vi "Connection.vi"(6 "Parameters":variant, 7 "Timeout":i32=5000, 8 "error in (no error)":errorcluster, 9 "Port":u16=102, 10 "IP Address":string, 11 "Simulated_PLC in":refnum<class "Simulated_PLC.lvclass">) -> (0 "error out":errorcluster, 3 "Simulated_PLC out":refnum<class "Simulated_PLC.lvclass">)   [LabVIEW 2025, in "Simulated_PLC.lvclass"]
uses:
  Simulated_PLC.lvclass
  PLC_Abstr/PLC_Abstr/PLC_Abstr.lvclass
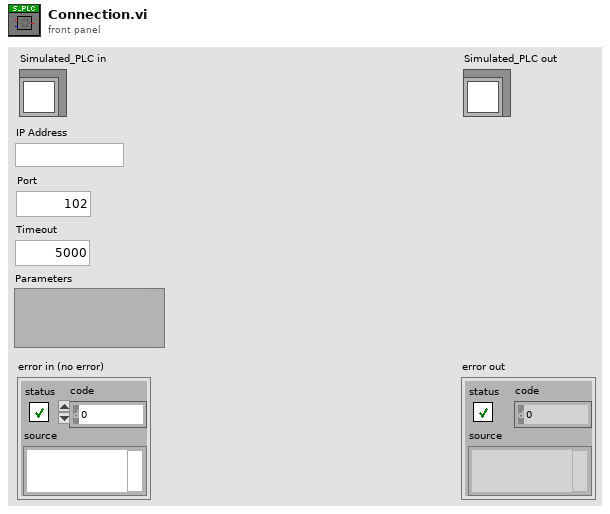
[diagram p1: front panel]
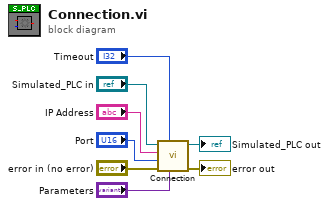
[diagram p0: block diagram]
diagram:
  n1 = call-parent "Connection.vi"("Parameters"="Parameters", "Timeout"="Timeout", "error in (no error)"="error in (no error)", "Port"="Port", "IP Address"="IP Address", "PLC_Abstr in"="Simulated_PLC in") -> ("error out"=→"error out":errorcluster, "PLC_Abstr out"=→"Simulated_PLC out":refnum<class "Simulated_PLC.lvclass">)  [unwired: 4 in]
